vi "Configure.vi"(8 "error in":errorcluster, 9 "Config Handle":T1, 10 "section":string="Serial Config", 11 "Serial Session in":refnum<class "Serial Session.lvclass">) -> (0 "error out":errorcluster, 3 "Serial Session out":refnum<class "Serial Session.lvclass">)   [LabVIEW 2019, in "Serial Session.lvclass"]
doc: "Configure uses an existing configuration file association to configure the port for operation."
uses:
  Serial Session.lvclass
  File Access/Config Data/Config Session.ctl
  File Access/Config Data/Config Data.lvclass
  Typedefs/Serial Config.ctl
  Typedefs/Msg Config.ctl
  File Access/Config Data/Config Data.lvclass/Config Data.ctl
  File Access/Config Data/Accessors/Read Ref.vi
  <vilib>/Utility/config.llb/Read Key (String).vi
  <vilib>/Utility/config.llb/NI_LVConfig.lvlib
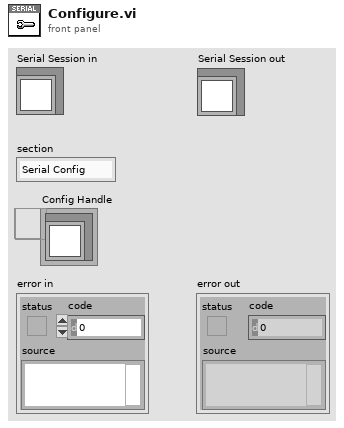
[diagram p1: front panel]
types:
  T1 = typedef "Config Data.lvclass/Config Session.ctl" = refnum<data-value>
  T2 = cluster{"EnTermChar":bool, "termChar":u8, "suppEnEnRd":bool, "sendEndEn":bool}
  T3 = typedef "Serial Session.lvclass/Msg Config.ctl" = cluster{"sendEndEn":bool, "suppEnEnRd":bool, "termChar":u8, "EnTermChar":bool}
  T4 = typedef "Serial Session.lvclass/Serial Config.ctl" = cluster{"baud rate":u32, "data bits":u16, "stop bits":u16, "parity":u16, "flow control":u16, "endModeforReads":u16, "endModeforWrites":u16}
  T5 = typedef "NI_LVConfig.lvlib/Config Data RefNum.ctl" = refnum<k1>
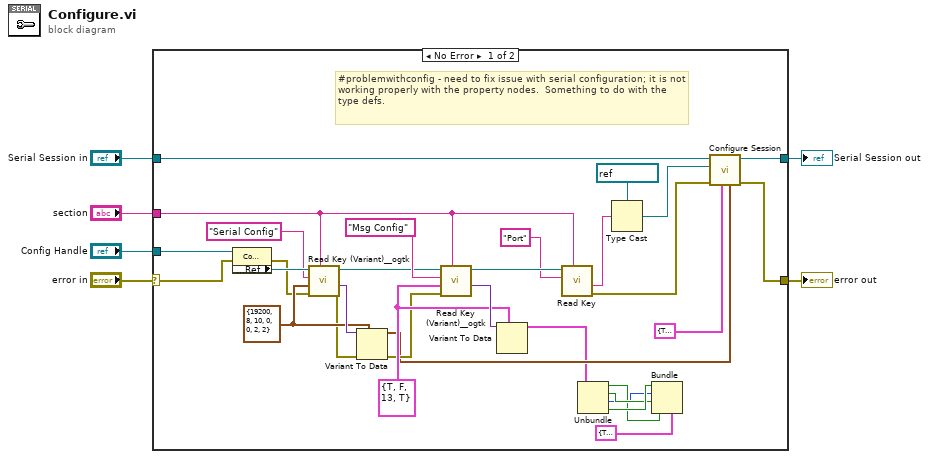
[diagram p0: block diagram]
diagram:
  n1 = case shown="No Error" "error in" {
    selector: "error in" -> [w24 w39]
    tunnel: [w15 w39] -> w5
    tunnel: [w18 w38] -> w3
    tunnel: "Serial Session in" -> [w19 w38]
    tunnel: "Config Handle" -> [w37 _]
    tunnel: "section" -> [w26 _]
    frame No Error {
      w29 = T3 {"sendEndEn"=TRUE, "suppEnEnRd"=FALSE, "termChar"=13, "EnTermChar"=TRUE} ("Msg Configuration")
      w34 = T4 {"baud rate"=19200, "data bits"=8, "stop bits"=10, "parity"=0, "flow control"=0, "endModeforReads"=2, "endModeforWrites"=2} ("Serial Config")
      # "#problemwithconfig - need to fix issue with serial configuration; it is not working properly with the property nodes.  Something to do with the type defs."
      n2 = property class="Config Data"(reference=w37, error in=w24) -> (error out=w23:errorcluster, "Accessors:Ref"=w36:T5)  [unwired: 1 out]
      n3 = call <userlib>:"Read Key (Variant)__ogtk.vi"("section"=w26, "error in (no error)"=w23, "type"=w34, "key (optional)"="Serial Config", "refnum"=w36) -> ("error out"=w33:errorcluster, "key-value"=w35:variant, "refnum out"=w22:T5)  [unwired: 3 in, 1 out]
      n4 = Variant To Data(error in=w33, type=w34, Variant=w35) -> (data=w14:T4, error out=w28:errorcluster)
      n5 = call <userlib>:"Read Key (Variant)__ogtk.vi"("section"=w26, "error in (no error)"=w28, "type"=w29, "key (optional)"="Msg Config", "refnum"=w22) -> ("key-value"=w30:variant, "refnum out"=w27:T5)  [unwired: 3 in, 2 out]
      n6 = Variant To Data(type=w29, Variant=w30) -> (data=w13:T3)  [unwired: 1 in, 1 out]
      n7 = call-poly <vilib>:"Read Key.vi"("section"=w26, "key"="Port", "refnum"=w27) -> ("error out"=w17:errorcluster, "value"=w21:string)  [unwired: 5 in, 2 out]
      n8 = Unbundle(w13) -> ("sendEndEn"=w9:bool, "suppEnEnRd"=w10:bool, "termChar"=w8:u8, "EnTermChar"=w11:bool)
      n9 = Type Cast(type=refnum<visa-resource-name> "COM5" ("VISA Resource"), x=w21) -> (*(type *) &x=w16:refnum<visa-resource-name>)
      n10 = Bundle(cluster=T2 {"EnTermChar"=TRUE, "termChar"=13, "suppEnEnRd"=FALSE, "sendEndEn"=TRUE} ("Message Cfg 2"), "EnTermChar"=w11, "termChar"=w8, "suppEnEnRd"=w10, "sendEndEn"=w9) -> ()  [unwired: 1 out]
      n11 = call "Configure Session.vi"("serialCfg"=w14, "Message Cfg"=T2 {"EnTermChar"=TRUE, "termChar"=13, "suppEnEnRd"=FALSE, "sendEndEn"=TRUE} ("Message Cfg 2"), "error in"=w17, "VISA Resource"=w16, "Serial Session"=w19) -> ("error out"=w15:errorcluster, "Serial Session out"=w18:refnum<class "Serial Session.lvclass">)  [unwired: 5 in]
    }
    frame Error {
    }
  }
  "error out" <- w5
  "Serial Session out" <- w3
